vi "IPC-Modbus-Transfer-EncodeResponse-ReadRegisters.vi"(11 "Register value":u16[](array[numeric])) -> (3 "输出字符串":string)   [LabVIEW 2014]
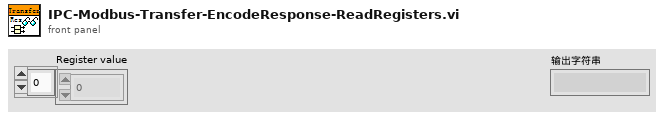
[diagram p1: front panel]
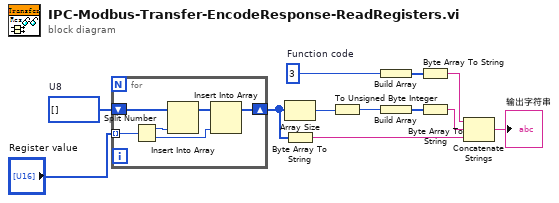
[diagram p0: block diagram]
diagram:
  w2 = u8[] []  # U8
  w11 = u8 3  # Function code
  n1 = for {
    tunnel: "Register value" -> [w18] mode=indexing
    shift-right: [w13] -> w1
    shift-left: w2 -> [w16]
    n2 = Split Number(x=w18) -> (hi(x)=w17:u8, lo(x)=w14:u8)
    n3 = Insert Into Array(array=w16, new element=w17) -> (w15:u8[])  [unwired: 1 in]
    n4 = Insert Into Array(array=w15, new element=w14) -> (w13:u8[])  [unwired: 1 in]
  }
  n5 = Array Size(array=w1) -> (size(s)=w3:i32)
  n6 = Byte Array To String(unsigned byte array=w1) -> (string=w7:string)
  n7 = To Unsigned Byte Integer(number=w3) -> (unsigned 8bit integer=w5:u8)
  n8 = Build Array(w11) -> (w12:u8[])
  n9 = Build Array(w5) -> (w10:u8[])
  n10 = Byte Array To String(unsigned byte array=w12) -> (string=w9:string)
  n11 = Byte Array To String(unsigned byte array=w10) -> (string=w8:string)
  n12 = Concatenate Strings(w9, w8, w7) -> (→"输出字符串":string)
